vi "stopkruispunt.vi"() -> ()   [LabVIEW 2019]
panel:
  in  "STOP kruispunt":bool
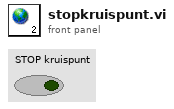
[diagram p1: front panel]
diagram:
